vi "Standalone_Nt_Client.vi"() -> ()   [LabVIEW 2025]
uses:
  <vilib>/Rock Robotics/Network Tables/NT Read Number.vi
  <vilib>/Rock Robotics/Network Tables/NT Write Number.vi
panel:
  out "Connected":bool
  out "Robot PV Loop Cnt":dbl
  out "LoopCount":dbl
  out "SetTeamError":errorcluster={"status"=FALSE, "code"=-1, "source"=""}
  out "error out":errorcluster={"status"=FALSE, "code"=-1, "source"=""}
  in  "TEAM":u64=4150
  in  "Client Name":string="VisionCoproc"
  in  "Update Time":i32=100
  # "Will return 0 if all is good"
  # "Team number."
  # "Arbitrary"
  # "Default"
  # "Can be faster."
  # "This was from the robot code I used for testing..."
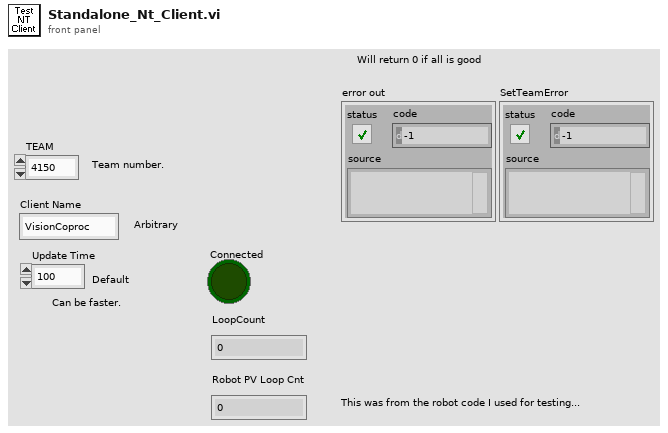
[diagram p1: front panel]
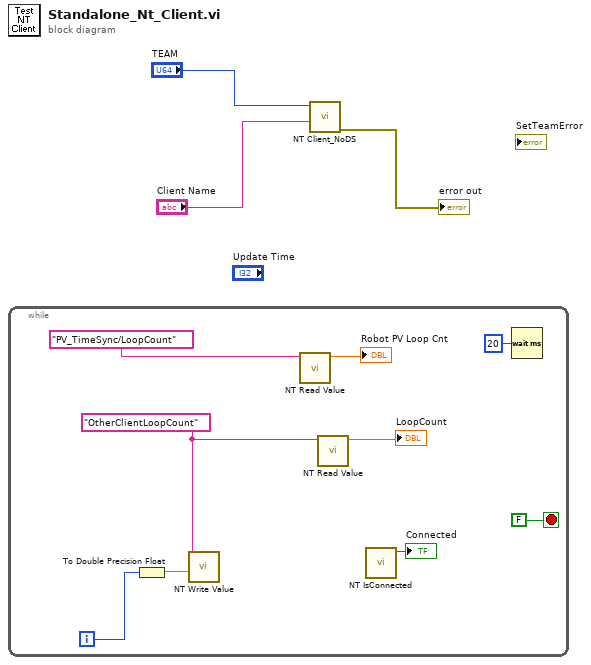
[diagram p0: block diagram]
diagram:
  n1 = while {
    i -> [w9]
    stop <- FALSE stop-if-true
    w8 = "OtherClientLoopCount" ("name")
    n2 = To Double Precision Float(number=w9) -> (double precision float=w10:dbl)
    n3 = call-poly <vilib>:"NT Write Value.vi"("value"=w10, "name"=w8) -> ()  [unwired: 9 in, 1 out]
    n4 = call-poly <vilib>:"NT Read Value.vi"("name"="PV_TimeSync/LoopCount") -> ("value"=→"Robot PV Loop Cnt":dbl)  [unwired: 8 in, 2 out]
    n5 = call-poly <vilib>:"NT Read Value.vi"("name"=w8) -> ("value"=→"LoopCount":dbl)  [unwired: 8 in, 2 out]
    n6 = call "NT IsConnected.vi"() -> ("Connected"=→"Connected":bool)  [unwired: 10 in, 1 out]
    n7 = Wait (ms)(milliseconds to wait=u32 20) -> ()  [unwired: 1 out]
  }
  n8 = call "NT Client_NoDS.vi"("Client Name"="Client Name", "TEAM"="TEAM") -> ("error out"=→"error out":errorcluster)  [unwired: 9 in]
